vi "GEA2 Register for Events.vi"(0 "GEA2 Reference In":refnum<k24>, 11 "Error In":errorcluster) -> (4 "GEA2 Reference Out":refnum<k24>, 6 "GEA2 Event Registration":refnum<event-registration>, 15 "Error Out":errorcluster)   [LabVIEW 2016, in "GEA2_Toolkit.lvlib"]
doc: "This VI registers for events such that any messages that appear on the GEA2 bus trigger an event in LabVIEW. This event can be wired into an event structure and the message can be handled."
uses:
  library/GEA2_Toolkit.lvlib
  type defs/Data Out.ctl
  C:/Technology Lab/NI-2010/Trunk/Utility/LabVIEW GEA2 Toolkit v1.0.0.0/Appliance.NET/GeaCommunication.dll
  Appliance.NET/GeaCommunication.dll
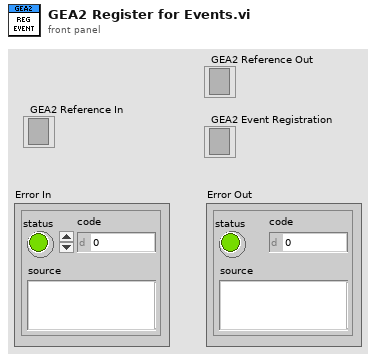
[diagram p1: front panel]
types:
  T1 = typedef "GEA2_Toolkit.lvlib/Data Out.ctl" = cluster{"Source":u8, "Destination":u8, "Command":u8, "Length":u8, "CRC":u16, "Message":string}
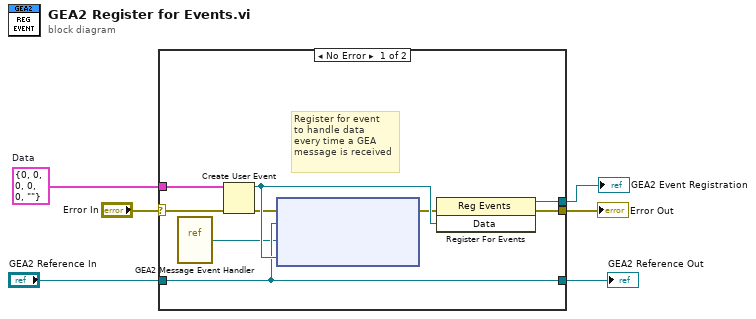
[diagram p0: block diagram]
diagram:
  w5 = T1 {"Source"=0, "Destination"=0, "Command"=0, "Length"=0, "CRC"=0, "Message"=""}  # Data
  n1 = case shown="No Error" "Error In" {
    selector: "Error In" -> [w8 w17]
    tunnel: [w14 w17] -> w6
    tunnel: w5 -> [w11 _]
    tunnel: [w10 _] -> w3
    tunnel: "GEA2 Reference In" -> [w9 w16]
    tunnel: [w9 w16] -> w2
    frame No Error {
      # "Register for event\nto handle data\nevery time a GEA\nmessage is received"
      n2 = vi-ref "GEA2 Message Event Handler.vi"() -> (w7:refnum<vi>)
      n3 = Create User Event(user event datatype=w11, error in=w8) -> (user event=w15:refnum<user-event>, error out=w13:errorcluster)
      n4 = node(w13, w9, w7, w15) -> (w12:errorcluster)  [unwired: 1 in, 1 out]
      n5 = register-events(error in=w12, w15) -> (reference out=w10:refnum<event-registration>, error out=w14:errorcluster)  [unwired: 1 in]
    }
    frame Error {
    }
  }
  "Error Out" <- w6
  "GEA2 Event Registration" <- w3
  "GEA2 Reference Out" <- w2
